vi "TimeConstant.vi"() -> ()   [LabVIEW 2021]
uses:
  <vilib>/Instr/_visa.llb/VISA Flush IO Buffer Mask.ctl
  <vilib>/Analysis/baseanly.llb/Mean (DBL).vi
  <vilib>/Instr/_visa.llb/VISA Configure Serial Port (Instr).vi
  <vilib>/measure/maspectr.llb/FFT Spectrum (Mag-Phase) for 1 Chan.vi
  <vilib>/measure/NI_MAPro.lvlib
  <vilib>/Analysis/NI_AALBase.lvlib
panel:
  out "Waveform Graph":cluster{"f0":dbl, "df":dbl, "magnitude":dbl[]}(graph)
  out "max value":dbl
  out "x+y":dbl
  out "max index(es)":i32
  out "x-y":dbl
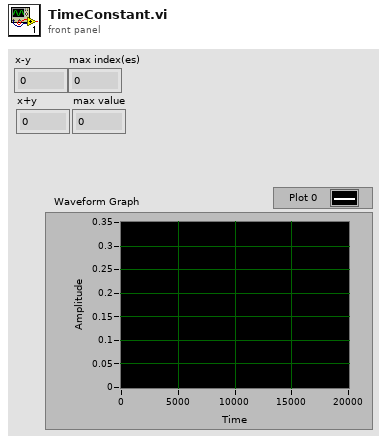
[diagram p1: front panel]
types:
  T1 = typedef "VISA Flush IO Buffer Mask.ctl" = u16
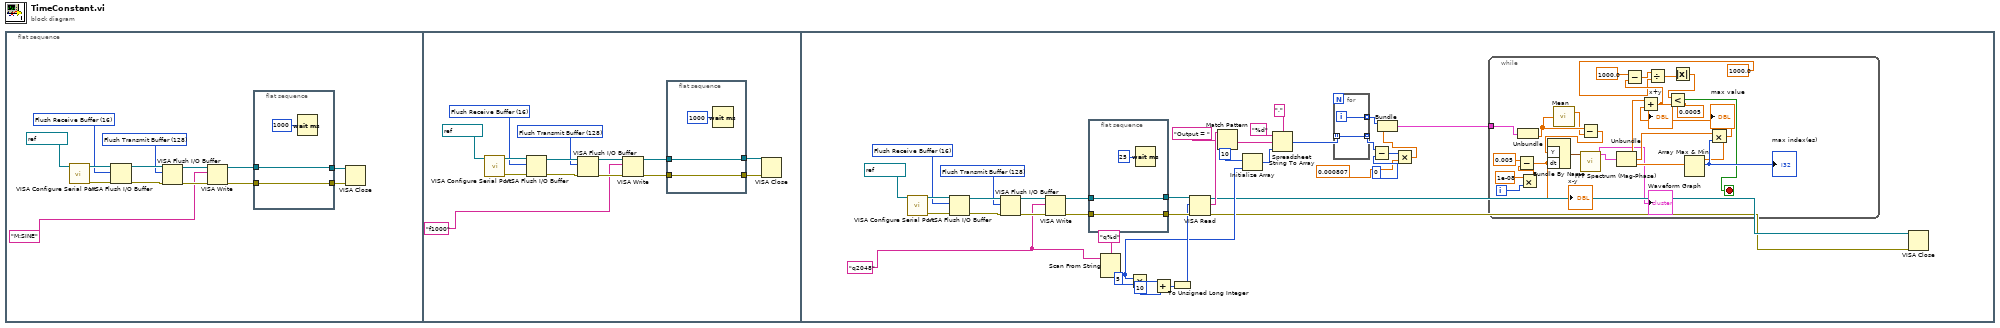
[diagram p0: block diagram]
diagram:
  n1 = flat-sequence {
    frame #0 {
      w8 = T1 128 items=["Flush Receive Buffer"=16, "Write Transmit Buffer to Device"=32, "Flush Receive Buffer (No I/O)"=64, "Flush Transmit Buffer"=128] ("Mask")
      w11 = T1 16 items=["Flush Receive Buffer"=16, "Write Transmit Buffer to Device"=32, "Flush Receive Buffer (No I/O)"=64, "Flush Transmit Buffer"=128] ("Mask")
      n2 = call-poly "VISA Configure Serial Port"("VISA resource name"=refnum<visa-resource-name> "COM5") -> ("VISA resource name out"=w13:refnum<visa-resource-name>, "error out"=w12:errorcluster)  [unwired: 13 in]
      n3 = VISA Flush I/O Buffer(VISA resource name=w13, mask (16)=w11, error in (no error)=w12) -> (VISA resource name out=w10:refnum<visa-resource-name>, error out=w9:errorcluster)
      n4 = VISA Flush I/O Buffer(VISA resource name=w10, mask (16)=w8, error in (no error)=w9) -> (VISA resource name out=w7:refnum<visa-resource-name>, error out=w6:errorcluster)
      n5 = VISA Write(VISA resource name=w7, write buffer="M:SINE", error in (no error)=w6) -> (VISA resource name out=w4:refnum<visa-resource-name>, error out=w2:errorcluster)  [unwired: 1 out]
      n6 = flat-sequence {
        tunnel: [w16] -> w3
        tunnel: w4 -> [w16]
        tunnel: w2 -> [w15]
        tunnel: [w15] -> w1
        frame #0 {
          n7 = Wait (ms)(milliseconds to wait=u32 1000) -> ()  [unwired: 1 out]
        }
      }
      n8 = VISA Close(VISA resource name=w3, error in (no error)=w1) -> ()  [unwired: 1 out]
    }
    frame #1 {
      w25 = T1 128 items=["Flush Receive Buffer"=16, "Write Transmit Buffer to Device"=32, "Flush Receive Buffer (No I/O)"=64, "Flush Transmit Buffer"=128] ("Mask")
      w28 = T1 16 items=["Flush Receive Buffer"=16, "Write Transmit Buffer to Device"=32, "Flush Receive Buffer (No I/O)"=64, "Flush Transmit Buffer"=128] ("Mask")
      n9 = call-poly "VISA Configure Serial Port"("VISA resource name"=refnum<visa-resource-name> "COM5") -> ("VISA resource name out"=w30:refnum<visa-resource-name>, "error out"=w29:errorcluster)  [unwired: 13 in]
      n10 = VISA Flush I/O Buffer(VISA resource name=w30, mask (16)=w28, error in (no error)=w29) -> (VISA resource name out=w27:refnum<visa-resource-name>, error out=w26:errorcluster)
      n11 = VISA Flush I/O Buffer(VISA resource name=w27, mask (16)=w25, error in (no error)=w26) -> (VISA resource name out=w24:refnum<visa-resource-name>, error out=w23:errorcluster)
      n12 = VISA Write(VISA resource name=w24, write buffer="f1000", error in (no error)=w23) -> (VISA resource name out=w22:refnum<visa-resource-name>, error out=w21:errorcluster)  [unwired: 1 out]
      n13 = flat-sequence {
        tunnel: [w34] -> w19
        tunnel: w22 -> [w34]
        tunnel: [w33] -> w18
        tunnel: w21 -> [w33]
        frame #0 {
          n14 = Wait (ms)(milliseconds to wait=u32 1000) -> ()  [unwired: 1 out]
        }
      }
      n15 = VISA Close(VISA resource name=w19, error in (no error)=w18) -> ()  [unwired: 1 out]
    }
    frame #2 {
      w35 = "q2048"
      w66 = T1 128 items=["Flush Receive Buffer"=16, "Write Transmit Buffer to Device"=32, "Flush Receive Buffer (No I/O)"=64, "Flush Transmit Buffer"=128] ("Mask")
      w69 = T1 16 items=["Flush Receive Buffer"=16, "Write Transmit Buffer to Device"=32, "Flush Receive Buffer (No I/O)"=64, "Flush Transmit Buffer"=128] ("Mask")
      n16 = call-poly "VISA Configure Serial Port"("VISA resource name"=refnum<visa-resource-name> "COM5") -> ("VISA resource name out"=w71:refnum<visa-resource-name>, "error out"=w70:errorcluster)  [unwired: 13 in]
      n17 = VISA Flush I/O Buffer(VISA resource name=w71, mask (16)=w69, error in (no error)=w70) -> (VISA resource name out=w68:refnum<visa-resource-name>, error out=w67:errorcluster)
      n18 = VISA Flush I/O Buffer(VISA resource name=w68, mask (16)=w66, error in (no error)=w67) -> (VISA resource name out=w65:refnum<visa-resource-name>, error out=w64:errorcluster)
      n19 = VISA Write(VISA resource name=w65, write buffer=w35, error in (no error)=w64) -> (VISA resource name out=w63:refnum<visa-resource-name>, error out=w62:errorcluster)  [unwired: 1 out]
      n20 = flat-sequence {
        tunnel: [w102] -> w61
        tunnel: w63 -> [w102]
        tunnel: [w101] -> w60
        tunnel: w62 -> [w101]
        frame #0 {
          n21 = Wait (ms)(milliseconds to wait=u32 25) -> ()  [unwired: 1 out]
        }
      }
      n22 = Scan From String(format string="q%d", input string=w35) -> (output 1=w47:i32)  [unwired: 3 in, 3 out]
      n23 = Multiply(x=w47, y=5) -> (x*y=w57:i32)
      n24 = Add(x=w57, y=10) -> (x+y=w55:i32)
      n25 = To Unsigned Long Integer(number=w55) -> (unsigned 32bit integer=w54:u32)
      n26 = VISA Read(VISA resource name=w61, byte count=w54, error in (no error)=w60) -> (VISA resource name out=w37:refnum<visa-resource-name>, read buffer=w53:string, error out=w36:errorcluster)  [unwired: 1 out]
      n27 = Match Pattern(string=w53, regular expression="Output = ") -> (after substring=w51:string)  [unwired: 1 in, 3 out]
      n28 = Initialize Array(10 ("y"), w47) -> (w46:i32[])
      n29 = Spreadsheet String To Array(delimiter (Tab)=",", format string="%d", spreadsheet string=w51, array type (2D Dbl)=w46) -> (array=w45:i32[])
      n30 = for {
        tunnel: w45 -> [w99] mode=indexing
        tunnel: [w99] -> w42 mode=indexing
        tunnel: [w98] -> w44 mode=indexing
        i -> [w98]
      }
      n31 = Subtract(x=w42, y=0) -> (x-y=w41:i32[])
      n32 = Multiply(x=w41, y=0.000807) -> (x*y=w39:dbl[])
      n33 = Bundle(w44, w39) -> (w38:cluster{i32[], dbl[]})  [unwired: 1 in]
      n34 = while {
        tunnel: w38 -> [w97]
        i -> [w94]
        stop <- w79 stop-if-true
        n35 = Unbundle(w97) -> (w75:dbl[])  [unwired: 1 out]
        n36 = Multiply(x=1e-08, y=w94) -> (x*y=w92:dbl)
        n37 = Subtract(x=0.005, y=w92) -> (x-y=w96:dbl)
        "x-y" <- w96
        n38 = call-poly <vilib>:"Mean.vi"("X"=w75) -> ("mean"=w74:dbl)  [unwired: 1 out]
        n39 = Subtract(x=w75, y=w74) -> (x-y=w73:dbl[])
        n40 = Bundle By Name("Y"=w73, "dt"=w96) -> (w91:waveform(dbl))  [unwired: 1 in]
        n41 = call-poly <vilib>:"FFT Spectrum (Mag-Phase).vi"("time signal"=w91) -> ("magnitude"=w76:cluster{"f0":dbl, "df":dbl, "magnitude":dbl[]})  [unwired: 6 in, 4 out]
        "Waveform Graph" <- w76
        n42 = Unbundle(w76) -> ("f0"=w88:dbl, "df"=w89:dbl, "magnitude"=w78:dbl[])
        n43 = Array Max & Min(array=w78) -> (max value=→"max value":dbl, max index (indices)=w90:i32)  [unwired: 2 out]
        "max index(es)" <- w90
        n44 = Multiply(x=w89, y=w90) -> (x*y=w87:dbl)
        n45 = Add(x=w88, y=w87) -> (x+y=w86:dbl)
        "x+y" <- w86
        n46 = Subtract(x=1000.0, y=w86) -> (x-y=w84:dbl)
        n47 = Divide(x=w84, y=1000.0) -> (x/y=w82:dbl)
        n48 = Absolute Value(x=w82) -> (abs(x)=w81:dbl)
        n49 = Less?(x=w81, y=0.0005) -> (x < y?=w79:bool)
      }
      n50 = VISA Close(VISA resource name=w37, error in (no error)=w36) -> ()  [unwired: 1 out]
    }
  }
